vi "Process File.vi"() -> ()   [LabVIEW 2019]
uses:
  <vilib>/Analysis/1siggen.llb/Ramp Pattern by Samples.vi
  <vilib>/Analysis/baseanly.llb/Mean (DBL).vi
  <vilib>/Analysis/1siggen.llb/Ramp Pattern by Delta.vi
  <vilib>/Analysis/2dsp.llb/1D Cross Correlation (DBL).vi
  <vilib>/Analysis/NI_AALPro.lvlib
  <vilib>/Analysis/NI_AALBase.lvlib
panel:
  out "Intensity Graph":dbl[][](graph)
  out "x = y?":bool
  out "Event Count Pairs":T1(array[cluster])
  out "Master Coincidence Indices":i32[](array[numeric])
  out "Minimum point":T2
  out "dt_m":i32[](array[numeric])
  out "dt_sc":i32[](array[numeric])
  out "max index(es)":i32
  out "Waveform Graph":dbl[](graph)
  out "Coincident Points":i32
  out "Master Points":i32
  out "size(s)":i32
  out "S-C Times":i32[](array[numeric])
  out "Master Times":i32[](array[numeric])
  out "XY Graph":cluster{cluster{i32, i32}[]}[](graph)
  out "Coincident Slave Points":cluster{"Numeric":i32, "Numeric":i32}[](array[cluster])
  out "S-S":cluster{"Numeric":i32, "Numeric":i32}[](array[cluster])
  out "Master Points":cluster{"Numeric":i32, "Numeric":i32}[](array[cluster])
  out "array":string[][](array[string])
  in  "Array":dbl[](array[numeric])
  # "date, time, count, time, adc, eventtype, deadtime, temp, name"
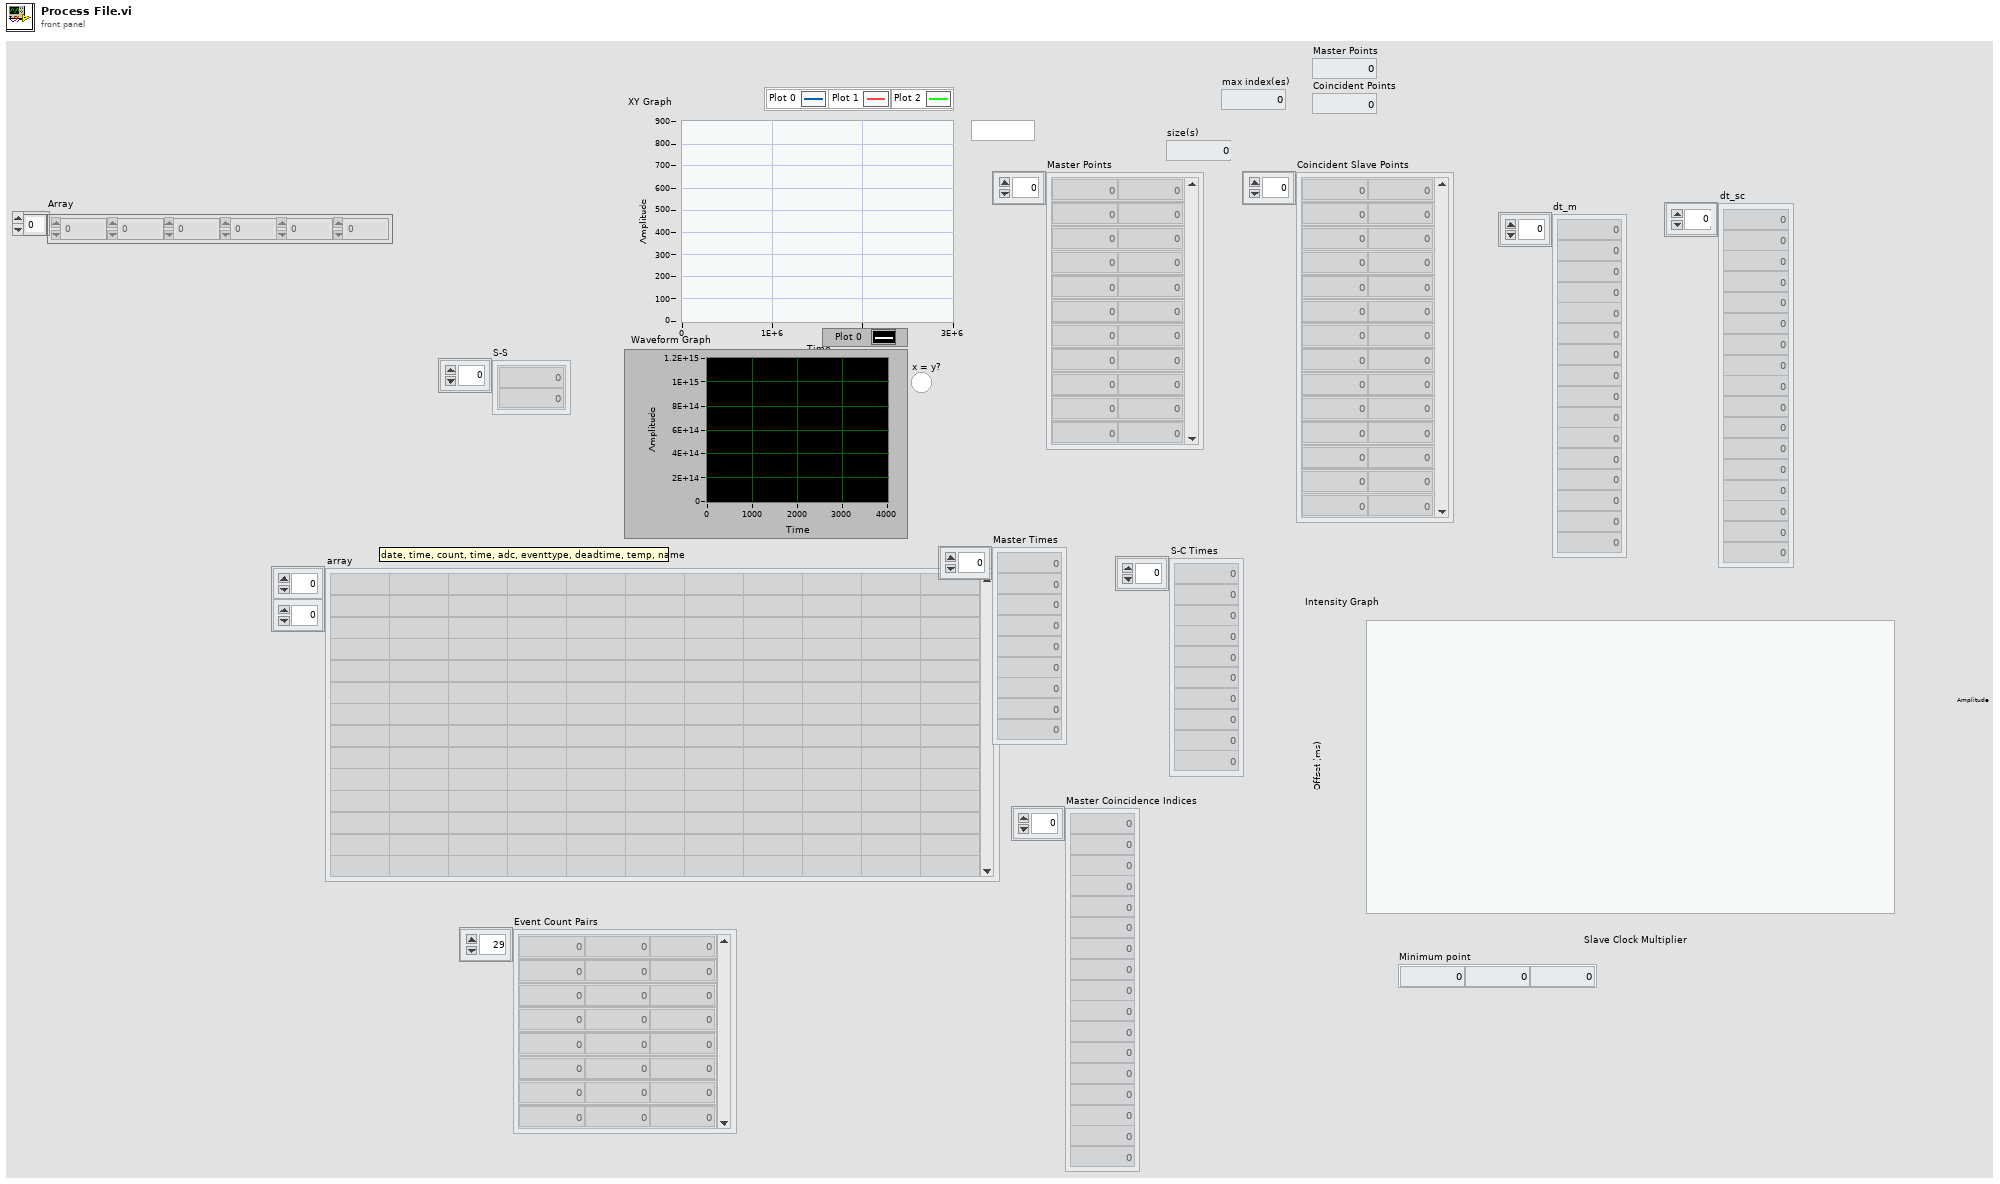
[diagram p1: front panel]
types:
  T1 = cluster{"Numeric":i32, "Numeric":i32, "Numeric 2":i32}[]
  T2 = cluster{"Numeric":dbl, "Numeric":dbl, "Numeric 2":dbl}
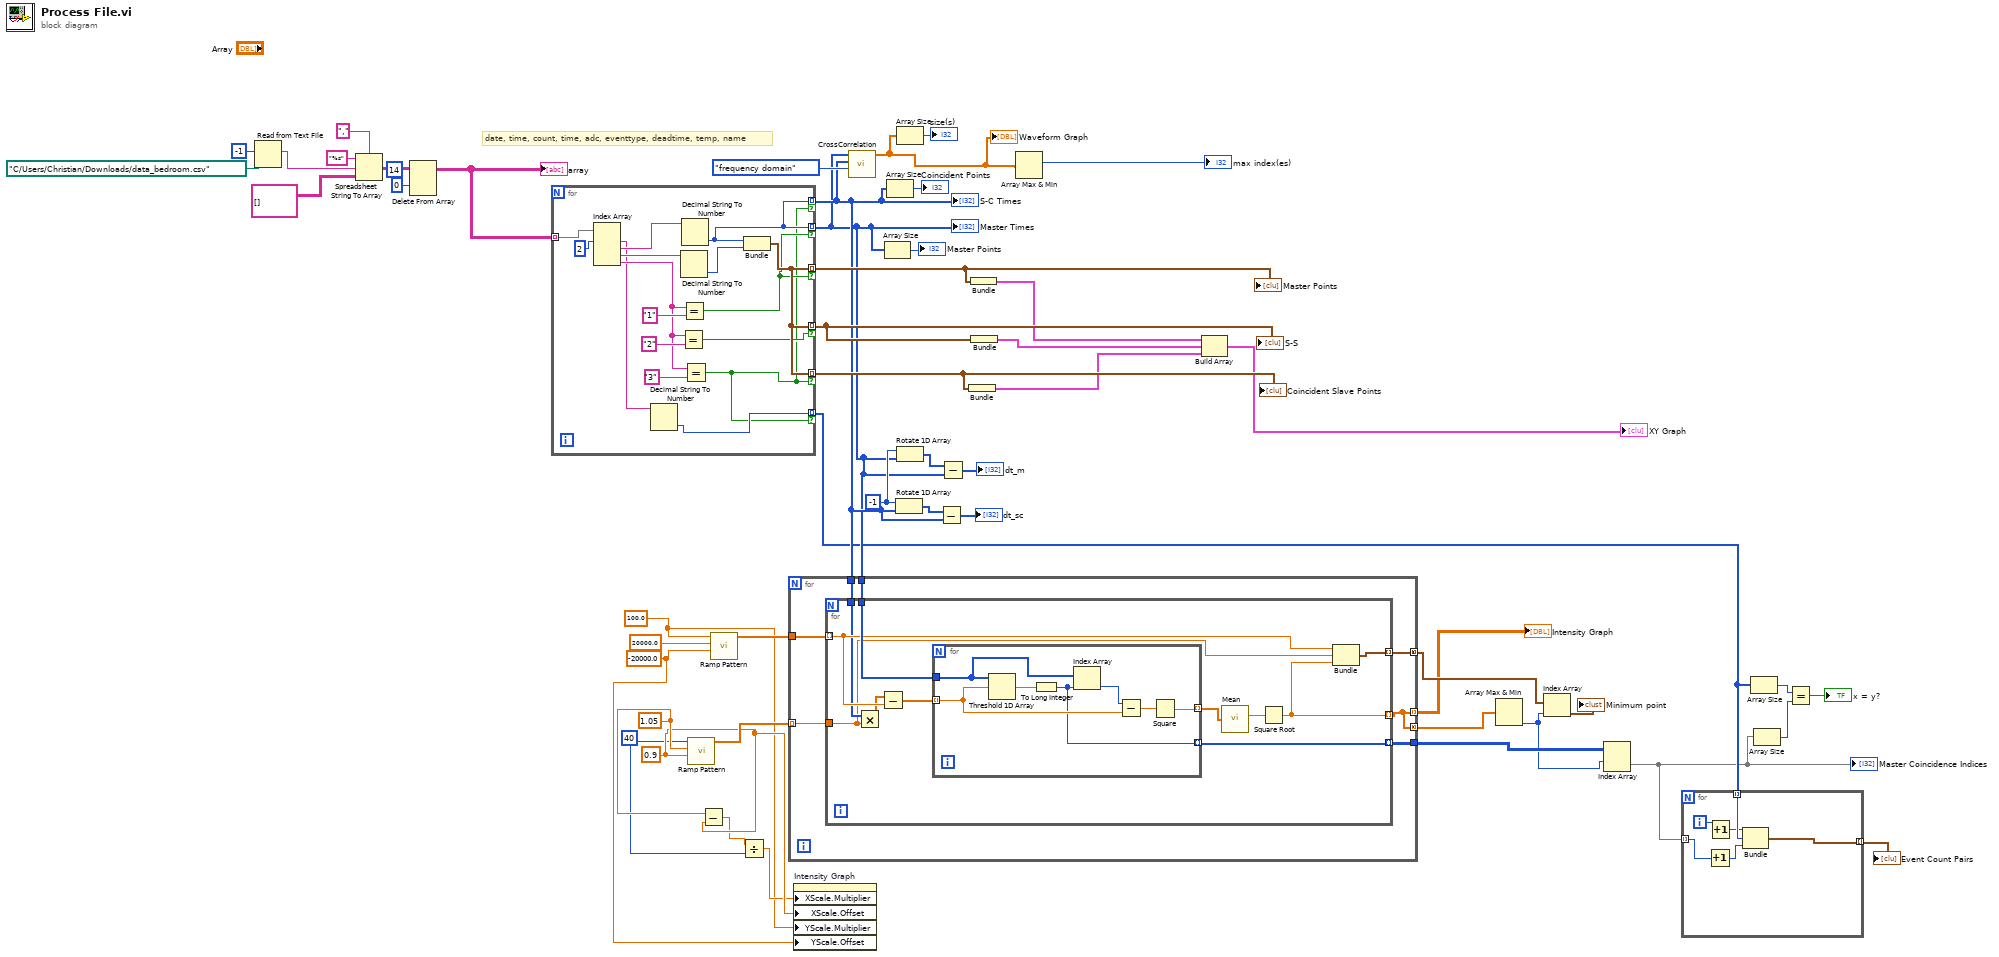
[diagram p0: block diagram]
diagram:
  w4 = 40 ("samples")
  w6 = 0.9 ("start")
  w7 = 1.05 ("end")
  w2 = -20000.0 ("start")
  w1 = 100.0 ("delta")
  w33 = -1 ("n")
  # "date, time, count, time, adc, eventtype, deadtime, temp, name"
  n1 = Read from Text File(file (use dialog)=path "C:/Users/Christian/Downloads/data_bedroom.csv", count=-1) -> (text=w14:string)  [unwired: 2 in, 3 out]
  n2 = Spreadsheet String To Array(delimiter (Tab)=",", format string="%s", spreadsheet string=w14, array type (2D Dbl)=string[][] []) -> (array=w50:string[][])
  n3 = Delete From Array(array=w50, length=14, index (row)=0) -> (array with subset deleted=w49:string[][])  [unwired: 1 in, 1 out]
  "array" <- w49
  n4 = for {
    tunnel: w49 -> [w61] mode=indexing
    tunnel: [w62] -> w46 mode=indexing if=w59
    tunnel: [w62] -> w45 mode=indexing if=w57
    tunnel: [w62] -> w44 mode=indexing if=w53
    tunnel: [w58] -> w27 mode=indexing if=w59
    tunnel: [w58] -> w28 mode=indexing if=w53
    tunnel: [w54] -> w19 mode=indexing if=w53
    n5 = Index Array(array=w61, index #1=2 ("index")) -> (element #1=w55:string, element #2=w65:string, element #3=w64:string, element #4=w60:string)  [unwired: 3 in]
    n6 = Decimal String To Number(string=w55) -> (number=w54:i32)  [unwired: 2 in, 1 out]
    n7 = Equal?(x=w60, y="2") -> (x = y?=w57:bool)
    n8 = Decimal String To Number(string=w64) -> (number=w63:i32)  [unwired: 2 in, 1 out]
    n9 = Equal?(x=w60, y="1") -> (x = y?=w59:bool)
    n10 = Decimal String To Number(string=w65) -> (number=w58:i32)  [unwired: 2 in, 1 out]
    n11 = Equal?(x=w60, y="3") -> (x = y?=w53:bool)
    n12 = Bundle(w58, w63) -> (w62:cluster{i32, i32})  [unwired: 1 in]
  }
  "Master Points" <- w46
  "S-S" <- w45
  "Coincident Slave Points" <- w44
  "Master Times" <- w27
  "S-C Times" <- w28
  n13 = call-poly <vilib>:"Ramp Pattern.vi"("start"=w6, "end"=w7, "samples"=w4) -> ("Ramp Pattern"=w10:dbl[])  [unwired: 7 in, 1 out]
  n14 = Subtract(x=w7, y=w6) -> (x-y=w5:dbl)
  n15 = call-poly <vilib>:"Ramp Pattern.vi"("start"=w2, "end"=20000.0, "delta"=w1) -> ("Ramp Pattern"=w25:dbl[])  [unwired: 6 in, 2 out]
  n16 = Divide(x=w5, y=w4) -> (x/y=w3:dbl)
  n17 = for {
    tunnel: w28 -> [w75]
    tunnel: w27 -> [w74]
    tunnel: w25 -> [w73]
    tunnel: [w69] -> w9 mode=indexing
    tunnel: [w72] -> w24 mode=concatenating
    tunnel: [w71] -> w22
    tunnel: w10 -> [w70] mode=indexing
    tunnel: [w69] -> w8 mode=concatenating
    n18 = for {
      tunnel: w75 -> [w78]
      tunnel: w74 -> [w86]
      tunnel: w73 -> [w82] mode=indexing
      tunnel: [w81] -> w72 mode=indexing
      tunnel: [w80] -> w69 mode=indexing
      tunnel: [w79] -> w71 mode=indexing
      tunnel: w70 -> [w76]
      n19 = Multiply(x=w78, y=w76) -> (x*y=w77:dbl[])
      n20 = Subtract(x=w77, y=w82) -> (x-y=w85:dbl[])
      n21 = for {
        tunnel: w85 -> [w90] mode=indexing
        tunnel: w86 -> [w92]
        tunnel: [w88] -> w84 mode=indexing
        tunnel: [w87] -> w79 mode=indexing
        n22 = Threshold 1D Array(2:w90, 3:w92) -> (0:w93:dbl)  [unwired: 1 in]
        n23 = To Long Integer(number=w93) -> (32bit integer=w87:i32)
        n24 = Index Array(array=w92, index=w87) -> (element=w91:i32)
        n25 = Subtract(x=w91, y=w90) -> (x-y=w89:dbl)
        n26 = Square(x=w89) -> (x^2=w88:dbl)
      }
      n27 = call-poly <vilib>:"Mean.vi"("X"=w84) -> ("mean"=w83:dbl)  [unwired: 1 out]
      n28 = Square Root(x=w83) -> (sqrt(x)=w80:dbl)
      n29 = Bundle(w82, w76, w80) -> (w81:cluster{dbl, dbl, dbl})  [unwired: 1 in]
    }
  }
  "Intensity Graph" <- w9
  n30 = property on="Intensity Graph" class="IntGraph (strict)"("XScale.Multiplier"=w3, "XScale.Offset"=w6, "YScale.Multiplier"=w1, "YScale.Offset"=w2) -> ()  [unwired: 2 in, 2 out]
  n31 = call-poly <vilib>:"CrossCorrelation.vi"("algorithm"=enum32{"direct", "frequency domain"}."frequency domain", "Y"=w28, "X"=w27) -> ("Rxy"=w35:dbl[])  [unwired: 7 in, 1 out]
  "Waveform Graph" <- w35
  n32 = Array Size(array=w27) -> (size(s)=→"Master Points":i32)
  n33 = Array Size(array=w28) -> (size(s)=→"Coincident Points":i32)
  n34 = Rotate 1D Array(1:w28, 2:w33) -> (0:w31:i32[])
  n35 = Array Size(array=w35) -> (size(s)=→"size(s)":i32)
  n36 = Rotate 1D Array(1:w27, 2:w33) -> (0:w32:i32[])
  n37 = Subtract(x=w31, y=w28) -> (x-y=→"dt_sc":i32[])
  n38 = Subtract(x=w32, y=w27) -> (x-y=→"dt_m":i32[])
  n39 = Bundle(w44) -> (w43:cluster{cluster{i32, i32}[]})  [unwired: 1 in]
  n40 = Bundle(w46) -> (w41:cluster{cluster{i32, i32}[]})  [unwired: 1 in]
  n41 = Bundle(w45) -> (w42:cluster{cluster{i32, i32}[]})  [unwired: 1 in]
  n42 = Array Max & Min(array=w35) -> (max index (indices)=→"max index(es)":i32)  [unwired: 3 out]
  n43 = Build Array(w41, w42, w43) -> (→"XY Graph":cluster{cluster{i32, i32}[]}[])
  n44 = Array Max & Min(array=w8) -> (min index (indices)=w21:i32)  [unwired: 3 out]
  n45 = Index Array(array=w24, index=w21) -> (element=→"Minimum point":cluster{dbl, dbl, dbl})
  n46 = Index Array(array=w22, index (row)=w21) -> (element=w18:i32[])  [unwired: 1 in]
  "Master Coincidence Indices" <- w18
  n47 = for {
    tunnel: w18 -> [w99] mode=indexing
    tunnel: [w97] -> w20 mode=indexing
    tunnel: w19 -> [w96] mode=indexing
    i -> [w95]
    n48 = Increment(x=w99) -> (x+1=w98:i32)
    n49 = Increment(x=w95) -> (x+1=w94:i32)
    n50 = Bundle(w94, w96, w98) -> (w97:cluster{i32, i32, i32})  [unwired: 1 in]
  }
  "Event Count Pairs" <- w20
  n51 = Array Size(array=w19) -> (size(s)=w17:i32)
  n52 = Array Size(array=w18) -> (size(s)=w16:i32)
  n53 = Equal?(x=w17, y=w16) -> (x = y?=→"x = y?":bool)
